vi "RichToFlatcif_manager_QueryPluginLoadersResponse.vi"(5 "OutputClusterType":T1, 11 "InputCluster":T4) -> (3 "OutputCluster":T1)   [LabVIEW 2021, in "CIF_PluginLoader_server.lvlib"]
uses:
  CIF_PluginLoader_server.lvlib
  cif_manager_QueryPluginLoadersResponse.ctl
  cif_manager_LoaderInfoFull.ctl
  cif_manager_LoaderType.ctl
  cif_manager_QueryPluginLoadersResponse_Flat.ctl
  cif_manager_LoaderInfoFull_Flat.ctl
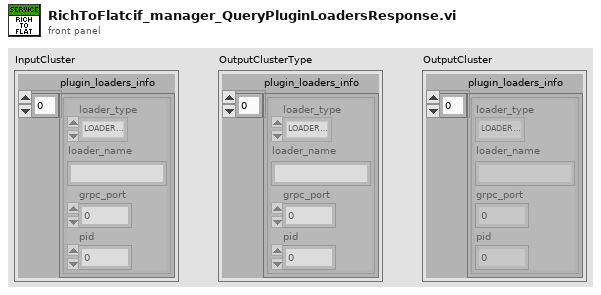
[diagram p1: front panel]
types:
  T1 = typedef "CIF_PluginLoader_server.lvlib/cif_manager_QueryPluginLoadersResponse_Flat.ctl" = cluster{"plugin_loaders_info":T2[]}
  T2 = typedef "CIF_PluginLoader_server.lvlib/cif_manager_LoaderInfoFull_Flat.ctl" = cluster{"loader_type":T3, "loader_name":string, "grpc_port":i32, "pid":u32}
  T3 = typedef "CIF_PluginLoader_server.lvlib/cif_manager_LoaderType.ctl" = enum32{"LOADERTYPE_UNKNOWN", "LOADERTYPE_LABVIEW"}
  T4 = typedef "CIF_PluginLoader_server.lvlib/cif_manager_QueryPluginLoadersResponse.ctl" = cluster{"plugin_loaders_info":T5[]}
  T5 = typedef "CIF_PluginLoader_server.lvlib/cif_manager_LoaderInfoFull.ctl" = cluster{"loader_type":T3, "loader_name":string, "grpc_port":i32, "pid":u32}
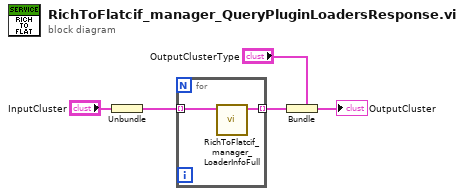
[diagram p0: block diagram]
diagram:
  n1 = Unbundle "Unbundle"("InputCluster") -> ("plugin_loaders_info"=w2:T5[])
  n2 = for {
    tunnel: w2 -> [w7] mode=indexing
    tunnel: [w6] -> w1 mode=indexing
    n3 = call "RichToFlatcif_manager_LoaderInfoFull.vi"("InputCluster"=w7) -> ("OutputCluster"=w6:T2)  [unwired: 10 in]
  }
  n4 = Bundle "Bundle"(cluster="OutputClusterType", "plugin_loaders_info"=w1) -> (→"OutputCluster":T1)
